vi "Test Process Request Returns when Process Stopped.vi"(8 "error in (no error)":errorcluster, 11 "Process Test In":refnum<class "Process Dev Test.lvclass">) -> (0 "error out":errorcluster, 3 "Process Test Out":refnum<class "Process Dev Test.lvclass">)   [LabVIEW 2020, in "Process Dev Test.lvclass"]
uses:
  Process Dev Test.lvclass
  C:/Program Files (x86)/National Instruments/LabVIEW 2020/vi.lib/Astemes/LUnit/Test Case.lvclass
  source/Framework Test Suite/Mock Process/Mock Process.lvclass
  C:/Git/astemes-triarc-framework/source/Framework/Process/Process.lvclass
  source/Framework/Process/Process.lvclass/Process.ctl
  <vilib>/Astemes/LUnit/Test Case.lvclass/Test Case.ctl
  <vilib>/Astemes/LUnit/LUnit Assertion Result.lvclass/LUnit Assertion Result.ctl
  <vilib>/Astemes/LUnit/LUnit Test Case Result.lvclass/LUnit Test Case Result.ctl
  <vilib>/Astemes/LUnit/LUnit Method Result.lvclass/LUnit Method Result.ctl
  source/Framework/Process/Private/SubVIs/Wait for finish.vi
  source/Framework/Process/Protected/Messaging/Enqueue Message.vi
  source/Framework/Process/Private/SubVIs/Set Lifecycle State.vi
  source/Framework/Process/Public/Lifecycle/Get Lifecycle State.vi
  <vilib>/Astemes/LUnit/Palette/Fail.vi
  <vilib>/Astemes/LUnit/Palette/Pass.vi
  <vilib>/Astemes/LUnit/Set Assertion Type.vi
  <vilib>/Astemes/LUnit/Palette/Pass If Equal.vi/cbf50e99-f124-4847-863a-8e9794d3dede.vi
  source/Framework/Process/Private/SubVIs/Handle Debug Data.vi
  <vilib>/Utility/error.llb/Clear Errors.vi
  <vilib>/Astemes/LUnit/Add test result.vi
  <vilib>/Astemes/LUnit/LUnit Write Passed.vi
  <vilib>/Astemes/LUnit/LUnit Write Message.vi
  <vilib>/Astemes/LUnit/LUnit Write Description.vi
  <vilib>/Astemes/LUnit/LUnit Write Assertion Type.vi
  <vilib>/Astemes/LUnit/Compare Variants.vi
  <vilib>/Astemes/LUnit/Describe Comparison.vi
  source/Framework/Logging/Log Debug.vi
  <vilib>/AdvancedString/1D String Array to Delimited String.vi
  <vilib>/Utility/High Resolution Relative Seconds.vi
  <vilib>/Astemes/LUnit/LUnit Record Assertion Result.vi
  <vilib>/Astemes/LUnit/Variant to string.vi
  <vilib>/Astemes/LUnit/LUnit Aggregate Assertion Results.vi
  <vilib>/Astemes/LUnit/Assertion Result/LUnit Read Status.vi
  <vilib>/Astemes/LUnit/LUnit Read Message.vi
  <vilib>/Astemes/LUnit/LUnit Read Description.vi
  <vilib>/Astemes/LUnit/Method Result/LUnit Merge Status.vi
  <vilib>/Astemes/LUnit/LUnit Concatenate result strings.vi
  <vilib>/Utility/error.llb/Error Cluster From Error Code.vi
  source/Framework/Process/Public/Read Name.vi
  <vilib>/Utility/Data Type/Get Type Information.vi
  <vilib>/Utility/LVClass/Get LV Class Name.vi
  <vilib>/Astemes/LUnit/LUnit Assertion Result.lvclass
  source/Framework/Process/Process.lvclass
  <vilib>/Astemes/LUnit/Test Case.lvclass
  source/Framework Test Suite/Support/Framework Test Support.lvlib
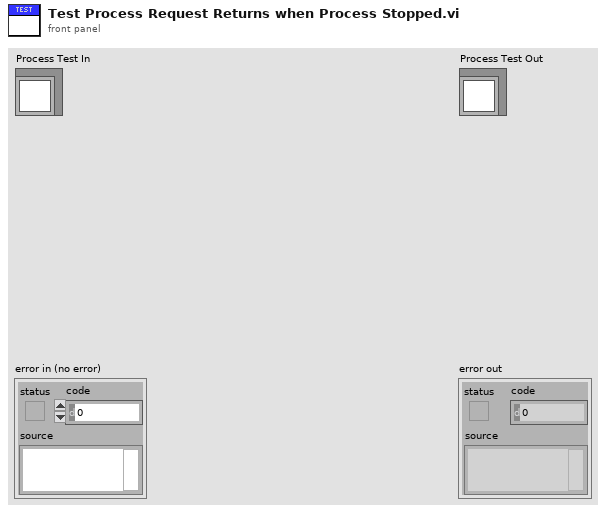
[diagram p1: front panel]
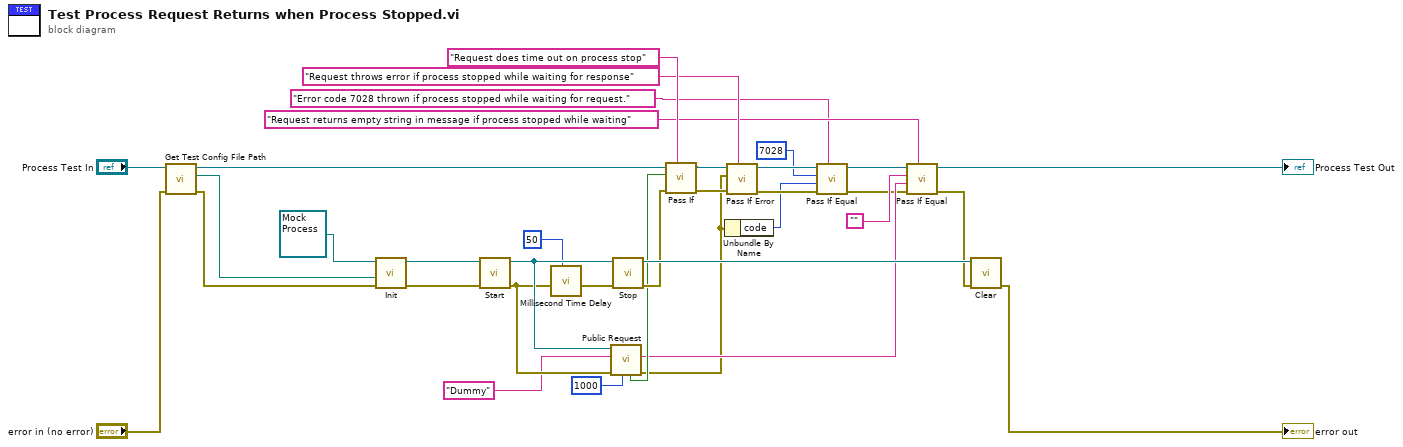
[diagram p0: block diagram]
diagram:
  n1 = call "Get Test Config File Path.vi"("error in (no error)"="error in (no error)", "Process Test In"="Process Test In") -> ("error out"=w27:errorcluster, "Test config path"=w28:path, "Process Test Out"=w30:refnum<class "Process Dev Test.lvclass">)  [unwired: 7 in]
  n2 = call-dynamic "Init.vi"("error in (no error)"=w27, "Config File Path"=w28, "Mock Process In"=refnum<class "Mock Process.lvclass"> refnum ("Mock Process.lvclass")) -> ("error out"=w31:errorcluster, "Mock Process Out"=w32:refnum<class "Mock Process.lvclass">)  [unwired: 7 in]
  n3 = call "Start.vi"("error in (no error)"=w31, "Process In"=w32) -> ("error out"=w22:errorcluster, "Process Out"=w23:refnum<class "Mock Process.lvclass">)  [unwired: 7 in, 1 out]
  n4 = call "Millisecond Time Delay.vi"("milliseconds to wait"=u32 50, "error in (no error)"=w22) -> ("error out"=w2:errorcluster)  [unwired: 7 in]
  n5 = call "Public Request.vi"("timeout in ms"=1000, "error in (no error)"=w22, "Request Message"="Dummy", "Mock Process In"=w23) -> ("error out"=w7:errorcluster, "Response Message"=w15:string, "Timed out?"=w20:bool)  [unwired: 3 in, 2 out]
  n6 = call "Stop.vi"("error in (no error)"=w2, "Process In"=w23) -> ("error out"=w34:errorcluster, "Process Out"=w35:refnum<class "Mock Process.lvclass">)  [unwired: 7 in, 1 out]
  n7 = call <vilib>:"Pass If.vi"("Description"="Request does time out on process stop", "error in (no error)"=w34, "Pass?"=w20, "LUnit Test Case In"=w30) -> ("error out"=w19:errorcluster, "LUnit Test Case Out"=w26:refnum<class "Process Dev Test.lvclass">)  [unwired: 6 in]
  n8 = Unbundle By Name(w7) -> ("code"=w6:i32)
  n9 = call <vilib>:"Pass If Error.vi"("Description"="Request throws error if process stopped while waiting for response", "error in (no error)"=w19, "Assert error"=w7, "LUnit Test Case In"=w26) -> ("error out"=w9:errorcluster, "LUnit Test Case Out"=w17:refnum<class "Process Dev Test.lvclass">)  [unwired: 6 in]
  n10 = call <vilib>:"Pass If Equal.vi"("Description"="Error code 7028 thrown if process stopped while waiting for request.", "error in (no error)"=w9, "Actual"=w6, "Expected"=7028 ("code"), "LUnit Test Case In"=w17) -> ("error out"=w8:errorcluster, "LUnit Test Case Out"=w10:refnum<class "Process Dev Test.lvclass">)  [unwired: 5 in]
  n11 = call <vilib>:"Pass If Equal.vi"("Description"="Request returns empty string in message if process stopped while waiting", "error in (no error)"=w8, "Actual"=w15, "Expected"="", "LUnit Test Case In"=w10) -> ("error out"=w18:errorcluster, "LUnit Test Case Out"=→"Process Test Out":refnum<class "Process Dev Test.lvclass">)  [unwired: 5 in]
  n12 = call-dynamic "Clear.vi"("error in (no error)"=w18, "Mock Process In"=w35) -> ("error out"=→"error out":errorcluster)  [unwired: 9 in]
